vi "SiosIfmGetPreset.vi"(1 "Channel":i32, 2 "Device Number":i32) -> (0 "Preset in nm":dbl)   [LabVIEW 2009]
uses:
  siosifm.dll
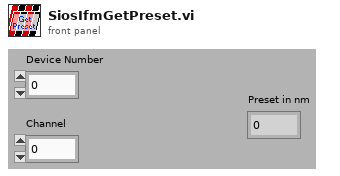
[diagram p1: front panel]
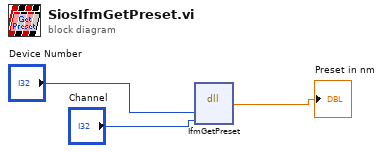
[diagram p0: block diagram]
diagram:
  n1 = dll-call lib="C:/WORK/Artem/RE-10/SIOS_IfmDLL/siosifm.dll" fn="IfmGetPreset"("devNumber"="Device Number", "Channel"="Channel") -> ("Preset"=→"Preset in nm":dbl)  [unwired: 5 in, 2 out]
